vi "Read configuration.vi"(8 "error in":errorcluster, 11 "Tank Controller Logic editor node in":refnum<class "Tank Controller Logic editor node.lvclass">) -> (0 "error out":errorcluster, 2 "configuration":refnum<class "NISE_CEF_serializable configuration.lvclass">, 3 "Tank Controller Logic editor node out":refnum<class "Tank Controller Logic editor node.lvclass">)   [LabVIEW 2017, in "Tank Controller Logic editor node.lvclass"]
uses:
  Tank Controller Logic editor node.lvclass
  <vilib>/NI/Configuration Framework/serializable configuration/NISE_CEF_serializable configuration.lvclass
  Tank Controller Logic editor node.lvclass/Tank Controller Logic editor node.ctl
  module/configuration/Tank Controller Logic configuration.lvclass
  C:/Program Files (x86)/National Instruments/LabVIEW 2017/vi.lib/NI/Configuration Framework/serializable configuration/NISE_CEF_serializable configuration.lvclass
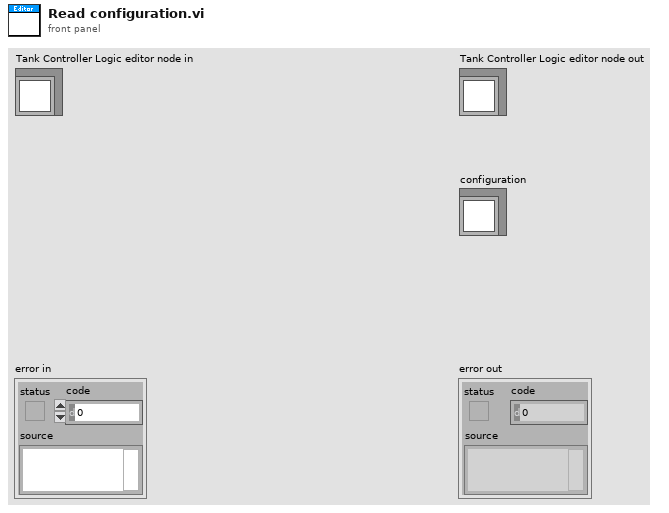
[diagram p1: front panel]
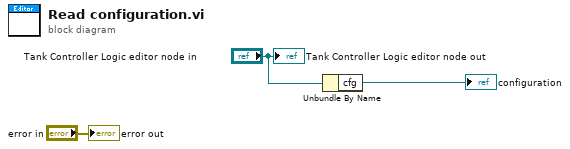
[diagram p0: block diagram]
diagram:
  n1 = Unbundle By Name("Tank Controller Logic editor node in") -> ("cfg"=→"configuration":refnum<class "Tank Controller Logic configuration.lvclass">)
  "error out" <- "error in"
  "Tank Controller Logic editor node out" <- "Tank Controller Logic editor node in"
